vi "Does File Exist.vi"(8 "error in (no error)":errorcluster, 9 "GUI helper Q":refnum<queue>, 10 "EMG Mode":bool=TRUE, 11 "GUI in":refnum<class "GUI.lvclass">) -> (0 "error out":errorcluster, 3 "GUI out":refnum<class "GUI.lvclass">)   [LabVIEW 2020, in "GUI.lvlib" / "GUI.lvclass"]
uses:
  GUI.lvclass
  C:/Program Files/National Instruments/LabVIEW 2020/vi.lib/ActorFramework/Actor/Actor.lvclass
  Task Active Enum df.ctl
  <vilib>/MGI/Panel Manager/Panel/Window Position/Reference Position/Alignment.ctl
  <vilib>/MGI/Panel Manager/Panel/Window Position/Reference Position/Horizontal Alignment.ctl
  <vilib>/MGI/Panel Manager/Panel/Window Position/Reference Position/Vertical Alignment.ctl
  GUI.lvclass/GUI.ctl
  Marker Enum.ctl
  <vilib>/ActorFramework/Actor/Actor.lvclass/Actor.ctl
  <vilib>/ActorFramework/Message Enqueuer/Message Enqueuer.lvclass/Message Enqueuer.ctl
  <vilib>/ActorFramework/Message Enqueuer/Init from Existing Queue.vi
  <vilib>/MGI/Panel Manager/Panel/Window Position/Reference Position/Ref Display/Ref Display.vi
  <vilib>/ActorFramework/Message Enqueuer/Message Enqueuer.lvclass
  <vilib>/MGI/Panel Manager/Panel/Panel.lvlib
  <vilib>/MGI/Panel Manager/Panel/Window Position/Reference Position/Reference Position.lvclass
  <vilib>/ActorFramework/Actor/Actor.lvclass
  GUI Messages/Accel Marker Update Msg/Accel Marker Update Msg.lvclass
  <vilib>/MGI/Panel Manager/Panel/Window Position/Reference Position/Ref Display/Ref Display.lvclass
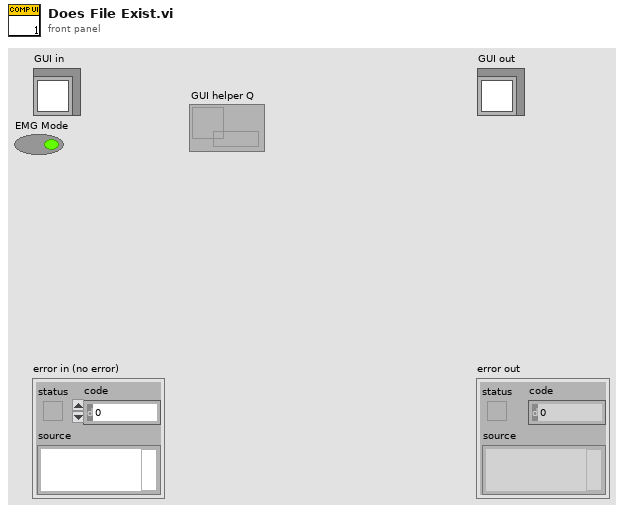
[diagram p1: front panel]
types:
  T1 = typedef "Panel.lvlib/Reference Position.lvclass/Alignment.ctl" = cluster{"Horizontal":T2, "Vertical":T3}
  T2 = typedef "Panel.lvlib/Reference Position.lvclass/Horizontal Alignment.ctl" = enum16{"Left", "Center", "Right"}
  T3 = typedef "Panel.lvlib/Reference Position.lvclass/Vertical Alignment.ctl" = enum16{"Top", "Center", "Bottom"}
  T4 = typedef "Marker Enum.ctl" = enum16{"Predefined", "Custom", "Delete Row", "Clear all"}
  T5 = typedef "Task Active Enum df.ctl" = enum16{"Idle", "Start Freq Task", "Start Freq Task and Accel", "Start Scanning Task", "Start Scanning Task and Accel", "Preview Template", "Collect MVC", "Calibrate Force", "Calibrate Potentiometers", "Stop Helper", "EMG Mode", "EMG and Accel Mode", "Task Config Update"}
  T6 = typedef "Subject and File df.ctl" = cluster{"File Save Path":path, "File Name ":string}
  T7 = typedef "Task selection df.ctl" = cluster{"Task Type Select":enum32{"Frequency Task", "Scanning Task"}, "Input Select Type":enum32{"Force Input", "Movement Input"}, "Collect EMG?":bool, "Collect acceleration?":bool, "EMG Rate":u16, "Acceleration Rate":u16}
  T8 = typedef "LVAllMonitorsDisplayTypeDef.ctl" = cluster{"Bounds":cluster{"Left":i16, "Top":i16, "Right":i16, "Bottom":i16}, "Depth":i16}[]
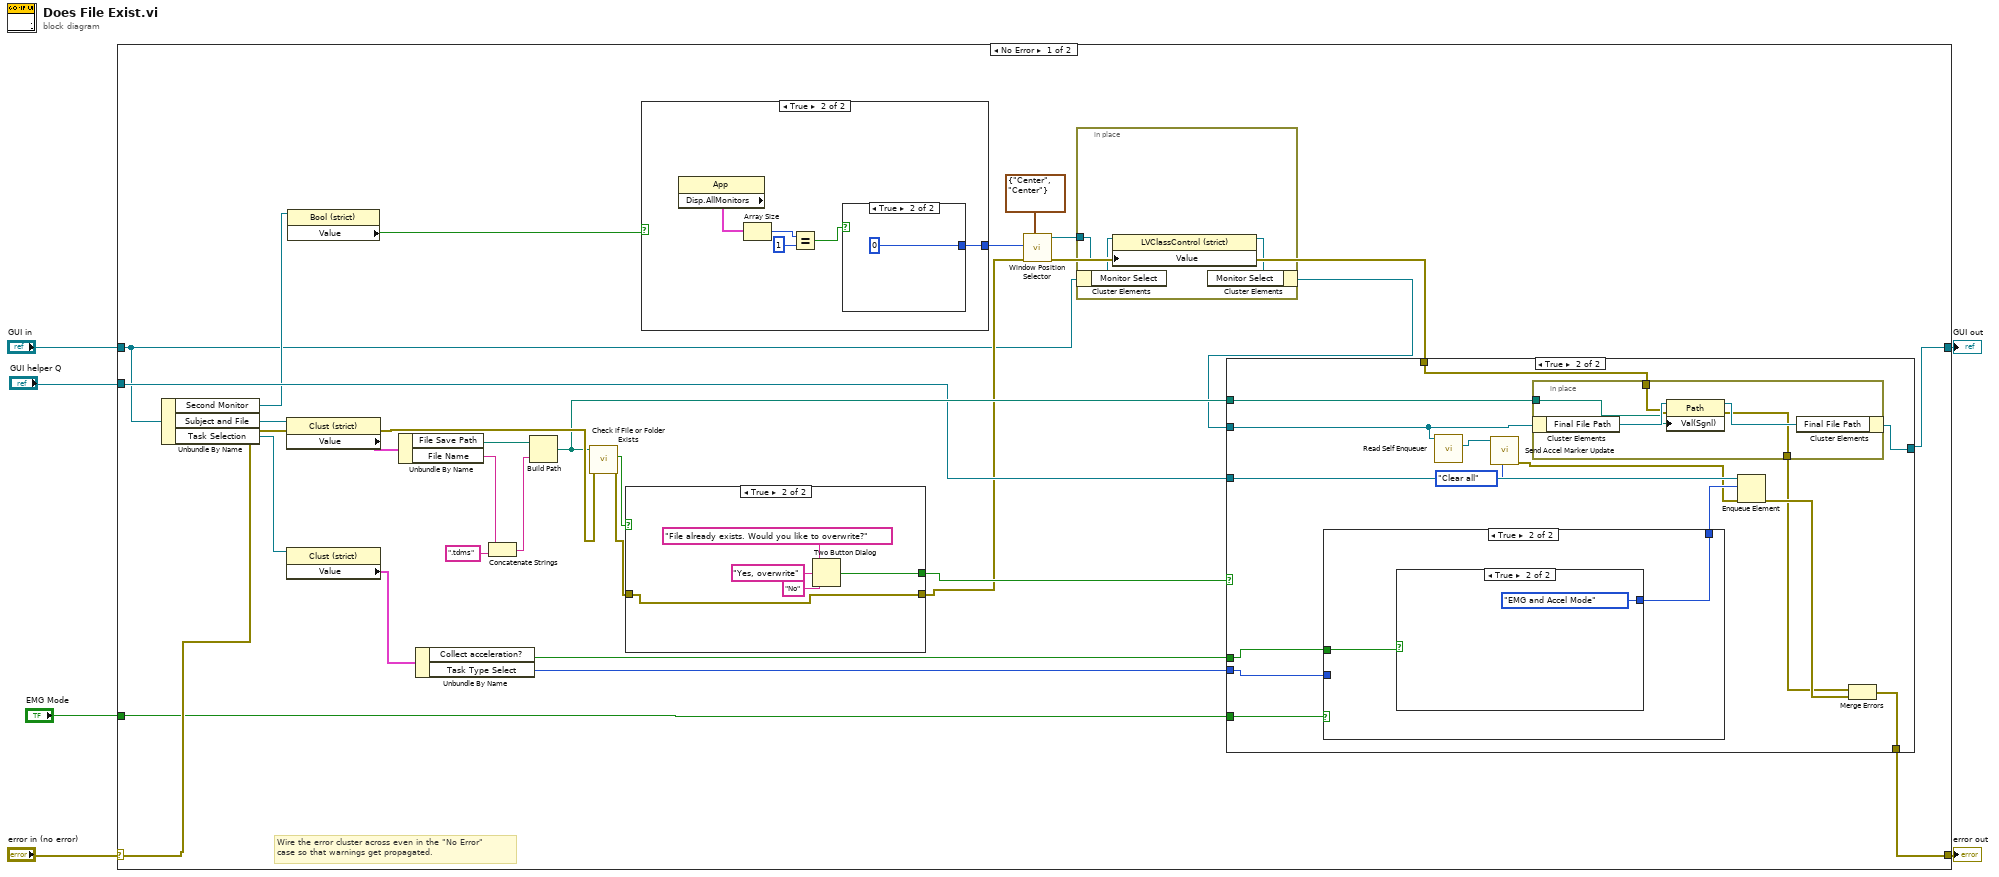
[diagram p0: block diagram]
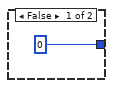
[diagram p2: hidden frame]
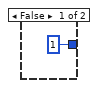
[diagram p3: hidden frame]
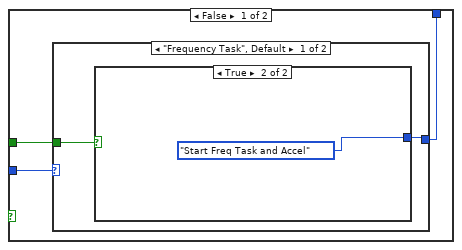
[diagram p5: hidden frame]
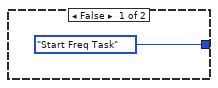
[diagram p6: hidden frame]
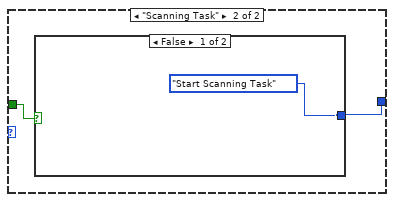
[diagram p7: hidden frame]
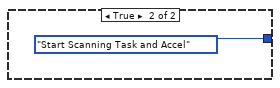
[diagram p8: hidden frame]
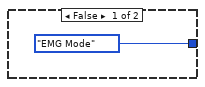
[diagram p9: hidden frame]
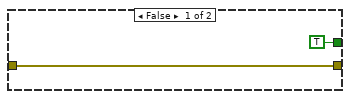
[diagram p10: hidden frame]
diagram:
  n1 = case shown="No Error" "error in (no error)" {
    selector: "error in (no error)" -> [w25 w92]
    tunnel: [w24 w92] -> w5
    tunnel: [w23 w91] -> w3
    tunnel: "GUI in" -> [w11 w91]
    tunnel: "GUI helper Q" -> [w21 _]
    tunnel: "EMG Mode" -> [w7 _]
    frame No Error {
      # "Wire the error cluster across even in the \"No Error\"\ncase so that warnings get propagated."
      n2 = Unbundle By Name(w11) -> ("Second Monitor"=w14:refnum<vi>, "Subject and File"=w35:refnum<vi>, "Task Selection"=w20:refnum<vi>)
      n3 = property class="Clust (strict)"(reference=w35, error in=w25) -> (error out=w29:errorcluster, "Value"=w34:T6)  [unwired: 1 out]
      n4 = property class="Clust (strict)"(reference=w20) -> ("Value"=w19:T7)  [unwired: 1 in, 2 out]
      n5 = property class="Bool (strict)"(reference=w14) -> ("Value"=w13:bool)  [unwired: 1 in, 2 out]
      n6 = Unbundle By Name(w34) -> ("File Save Path"=w33:path, "File Name"=w32:string)
      n7 = Unbundle By Name(w19) -> ("Collect acceleration?"=w18:bool, "Task Type Select"=w17:enum32{"Frequency Task", "Scanning Task"})
      n8 = Concatenate Strings(w32, ".tdms" ("string")) -> (w30:string)
      n9 = Build Path(base path=w33, name or relative path=w30) -> (appended path=w22:path)
      n10 = call <vilib>:"Check if File or Folder Exists.vi"("error in (no error)"=w29, "path"=w22) -> ("error out"=w26:errorcluster, "file or folder exists?"=w28:bool)  [unwired: 7 in, 1 out]
      n11 = case shown="True" w28 {
        tunnel: [TRUE ("T button?") w87] -> w27
        tunnel: w26 -> [w84 w86]
        tunnel: [w84 w86] -> w12
        frame False {
        }
        frame True {
          n12 = Two Button Dialog(message="File already exists. Would you like to overwrite?", 1:"No" ("F button name (\"Cancel\")"), 2:"Yes, overwrite" ("T button name (\"OK\")")) -> (T button?=w87:bool)
        }
      }
      n13 = case shown="True" w13 {
        tunnel: [0 ("Display (Primary)") w44] -> w16
        frame False {
        }
        frame True {
          n14 = property class="App"() -> ("Disp.AllMonitors"=w43:T8)  [unwired: 2 in, 2 out]
          n15 = Array Size(array=w43) -> (size(s)=w42:i32)
          n16 = Equal?(x=w42, y=1) -> (x = y?=w40:bool)
          n17 = case shown="True" w40 {
            tunnel: [1 ("Display (Primary)") 0 ("Display (Primary)")] -> w44
            frame False {
            }
            frame True {
            }
          }
        }
      }
      n18 = call-poly <vilib>:"Window Position Selector.vi"("Alignment"=T1 {"Horizontal"=enum."Center", "Vertical"=enum."Center"}, "Error In"=w12, "Display (Primary)"=w16) -> ("Error Out"=w8:errorcluster, "Ref Display out"=w10:refnum<class "Ref Display.lvclass">)  [unwired: 7 in]
      n19 = in-place {
        in-place-border: w10 -> [w37]
        n20 = in-place-cluster #1(w11) -> ("Monitor Select"=w36:refnum<vi>)
        n21 = property class="LVClassControl (strict)"(reference=w36, "Value"=w37) -> (reference out=w38:refnum<vi>)  [unwired: 1 in, 1 out]
        n22 = in-place-cluster #1("Monitor Select"=w38) -> (w9:refnum<class "GUI.lvclass">)
      }
      n23 = case shown="True" w27 {
        tunnel: [w47 w56] -> w24
        tunnel: [w48 w63] -> w23
        tunnel: w22 -> [_ w62]
        tunnel: w21 -> [_ w61]
        tunnel: w18 -> [_ w60]
        tunnel: w17 -> [_ w59]
        tunnel: w9 -> [w48 w54]
        tunnel: w8 -> [w47 w51]
        tunnel: w7 -> [_ w49]
        frame False {
        }
        frame True {
          n24 = case shown="True" w49 {
            tunnel: w60 -> [w66 w75]
            tunnel: w59 -> [w65 _]
            tunnel: [w64 w76] -> w58
            frame False {
              n25 = case shown="\"Frequency Task\", Default" w65 {
                tunnel: [w67 w71] -> w64
                tunnel: w66 -> [w68 w72]
                frame "Frequency Task", Default {
                  n26 = case shown="True" w68 {
                    tunnel: [Task_Active_Enum_df."Start Freq Task" ("element") Task_Active_Enum_df."Start Freq Task and Accel" ("element")] -> w67
                    frame False {
                    }
                    frame True {
                    }
                  }
                }
                frame "Scanning Task" {
                  n27 = case shown="False" w72 {
                    tunnel: [Task_Active_Enum_df."Start Scanning Task" ("element") Task_Active_Enum_df."Start Scanning Task and Accel" ("element")] -> w71
                    frame False {
                    }
                    frame True {
                    }
                  }
                }
              }
            }
            frame True {
              n28 = case shown="True" w75 {
                tunnel: [Task_Active_Enum_df."EMG Mode" ("element") Task_Active_Enum_df."EMG and Accel Mode" ("element")] -> w76
                frame False {
                }
                frame True {
                }
              }
            }
          }
          n29 = call <vilib>:"Read Self Enqueuer.vi"("Actor"=w54) -> ("Self Enqueuer"=w53:refnum<class "Message Enqueuer.lvclass">)  [unwired: 10 in]
          n30 = call "Send Accel Marker Update.vi"("Marker Enum"=Marker_Enum."Clear all", "Message Enqueuer in"=w53) -> ("error out"=w50:errorcluster)  [unwired: 8 in, 1 out]
          n31 = in-place {
            in-place-border: w62 -> [w81]
            in-place-border: [w80] -> w55
            in-place-border: w51 -> [w79]
            n32 = in-place-cluster #2(w54) -> ("Final File Path"=w83:refnum<vi>)
            n33 = property class="Path"(reference=w83, error in=w79, "Val(Sgnl)"=w81) -> (reference out=w82:refnum<vi>, error out=w80:errorcluster)
            n34 = in-place-cluster #2("Final File Path"=w82) -> (w63:refnum<class "GUI.lvclass">)
          }
          n35 = Enqueue Element(queue=w61, element=w58, error in (no error)=w50) -> (error out=w57:errorcluster)  [unwired: 1 in, 2 out]
          n36 = Merge Errors(w55, w57) -> (w56:errorcluster)
        }
      }
    }
    frame Error {
    }
  }
  "error out" <- w5
  "GUI out" <- w3
